vi "Left Flywheel Moter.vi"(8 "error in":errorcluster, 10 "Invert (default false)":bool, 11 "CAN Id":u8=3) -> (0 "error out":errorcluster)   [LabVIEW 2015]
uses:
  Support/Global Objects.vi
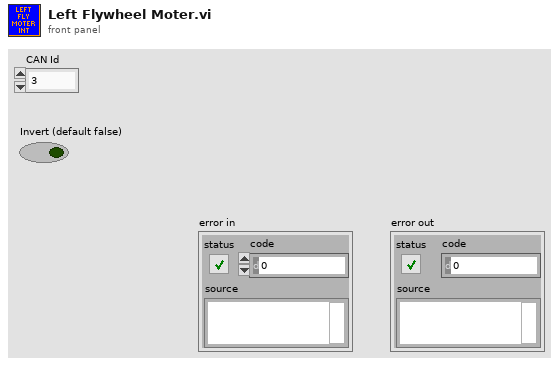
[diagram p1: front panel]
types:
  T1 = typedef "Motor Typedef.ctl" = cluster{"Motor1":T2, "Last Motor Power":dbl}
  T2 = typedef "WPI_MotorControlDeviceRef.ctl" = cluster{"DeviceStatus":errorcluster, "Type":T3, "PWM":cluster{"PWM Channel":T4, "DeadBand":T5}, "CAN":cluster{"Device Number":u8, "Control Mode":T6, "Semaphore":T7, "Max Vout":dbl, "TalonSRX Control Mode":T8}, "Invert":bool}
  T3 = typedef "WPI_MotorControlType.ctl" = enum16{"PWM", "CAN", "CANTalonSRX"}
  T4 = typedef "FPGA_DIOPWMChannel.ctl" = enum8{"PWM 0", "PWM 1", "PWM 2", "PWM 3", "PWM 4", "PWM 5", "PWM 6", "PWM 7", "PWM 8", "PWM 9", "PWM MXP 0", "PWM MXP 1", "PWM MXP 2", "PWM MXP 3", "PWM MXP 4", "PWM MXP 5", "PWM MXP 6", "PWM MXP 7", "PWM MXP 8", "PWM MXP 9", "Invalid"}
  T5 = typedef "WPI_PWMDeadband.ctl" = cluster{"Name":string, "maxPositivePwm":i32, "minPositivePwm":i32, "centerPwm":i32, "maxNegativePwm":i32, "minNegativePwm":i32, "angularRange":u16}
  T6 = typedef "WPI_CANJaguar_ControlMode.ctl" = enum8{"Percent VBus", "Current", "Speed", "Position", "Voltage"}
  T7 = typedef "Semaphore RefNum" = refnum<k1>
  T8 = typedef "WPI_CANTalonSRX_APIControlMode.ctl" = enum8{"Percent VBus", "Speed", "Position", "Slave", "Unchanged / Invalid", "Voltage Compensation", "Current", "Motion Profile"}
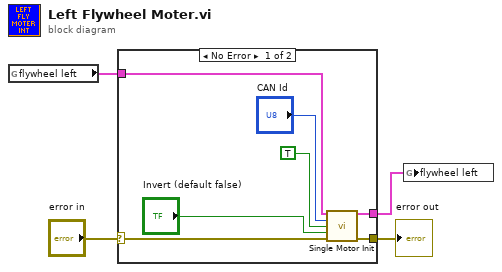
[diagram p0: block diagram]
diagram:
  n1 = global read "Global Objects.vi" "flywheel left"() -> (w2:T1)
  n2 = case shown="No Error" "error in" {
    selector: "error in" -> [w10 w13]
    tunnel: [w9 w13] -> w3
    tunnel: w2 -> [w6 w12]
    tunnel: [w11 w12] -> w1
    frame No Error {
      n3 = call "Single Motor Init.vi"("Motor In"=w6, "CAN Id"="CAN Id", "Use Can"=TRUE, "Invert (default false)"="Invert (default false)", "error in"=w10) -> ("Motor Out"=w11:T1, "error out"=w9:errorcluster)  [unwired: 9 in]
    }
    frame Error {
    }
  }
  "error out" <- w3
  n4 = global write "Global Objects.vi" "flywheel left"(w1) -> ()
